vi "Photocell Example.vi"() -> ()   [LabVIEW 2015, in "LabVIEW Interface for Arduino.lvlib"]
doc: "An example that uses the Arduino to read the value of a photocell."
uses:
  <vilib>/LabVIEW Interface for Arduino/LabVIEW Interface for Arduino.lvlib
  <vilib>/LabVIEW Interface for Arduino/Type Defs/Analog Pin.ctl
panel:
  in  "Stop":bool
  out "Light Intensity (0 - 100)":dbl(knob) scale=0.0..100.0
  in  "Photo Cell Pin (AI 0-5)":T1=enum."Anlog In 1"
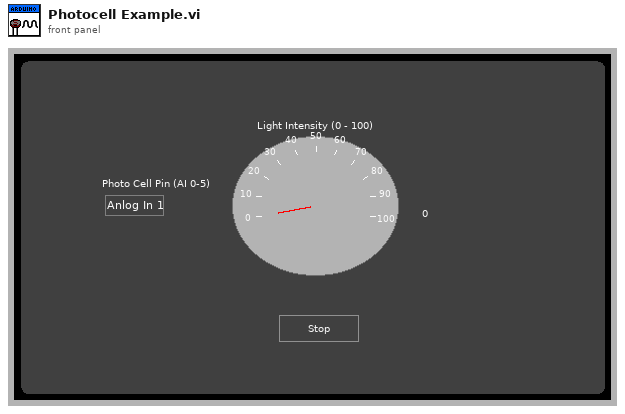
[diagram p1: front panel]
types:
  T1 = typedef "LabVIEW Interface for Arduino.lvlib/Analog Pin.ctl" = enum8{"Anlog In 0", "Anlog In 1", "Anlog In 2", "Anlog In 3", "Anlog In 4", "Anlog In 5"}
  T2 = typedef "LabVIEW Interface for Arduino.lvlib/Arduino Resource.ctl" = cluster{"VISA resource":refnum<visa-resource-name>, "Board Type":T3, "Connection Type":enum8{"USB / Serial"}, "Bytes Per Packet (15)":u8}
  T3 = typedef "LabVIEW Interface for Arduino.lvlib/Board Type.ctl" = enum16{"Uno", "Dimuelanove w/Atmega 328", "Mega 2560"}
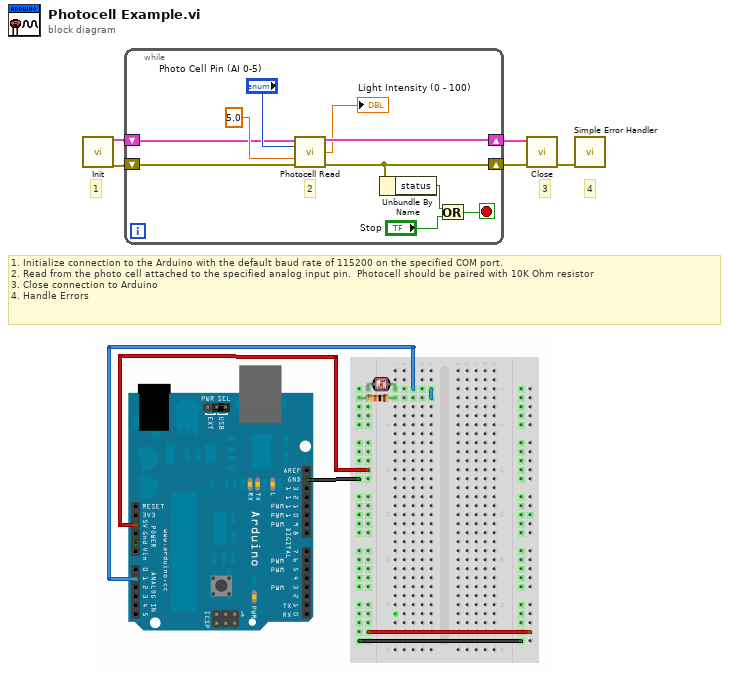
[diagram p0: block diagram]
diagram:
  # "1. Initialize connection to the Arduino with the default baud rate of 115200 on the specified COM port.\n2. Read from the photo cell attached to the specified analog input pin.  Photocell should be paired with 10K Ohm resistor\n3. Close connection to Arduino\n4. Handle Errors"
  # "4"
  # "3"
  # "1"
  n1 = call <vilib>:"Init.vi"() -> ("Arduino Resource"=w4:T2, "error out"=w3:errorcluster)  [unwired: 18 in]
  n2 = while {
    shift-right: [w10] -> w5
    shift-left: w3 -> [w15]
    shift-right: [w14] -> w1
    shift-left: w4 -> [w6]
    stop <- w7 stop-if-true
    # "2"
    n3 = call <vilib>:"Photocell Read.vi"("Arduino Resource"=w6, "Photo Cell Pin (0)"="Photo Cell Pin (AI 0-5)", "Vcc (5)"=5.0 ("Vcc"), "error in"=w15) -> ("Arduino Resource"=w14:T2, "Light Intensity (0 - 100)"=→"Light Intensity (0 - 100)":dbl, "error out"=w10:errorcluster)  [unwired: 9 in]
    n4 = Unbundle By Name(w10) -> ("status"=w9:bool)
    n5 = Or(x=w9, y="Stop") -> (x .or. y?=w7:bool)
  }
  n6 = call <vilib>:"Close.vi"("Arduino Resource"=w1, "error in"=w5) -> ("error out"=w2:errorcluster)  [unwired: 13 in]
  n7 = call <vilib>:"Simple Error Handler.vi"("error in (no error)"=w2) -> ()  [unwired: 4 in, 5 out]
